vi "Stratified KFold Indices.vi"(8 "error in (no error)":errorcluster, 9 "seed":i32=-1 caption="seed (-1)", 10 "Nr Folds":i32=10 caption="Nr Folds (10)", 11 "Labels y":dbl[](array[numeric])) -> (0 "error out":errorcluster, 3 "Stratified KFold indices":cluster{"elements":i32[]}[](array[cluster]))   [LabVIEW 2014]
uses:
  <userlib>/_OpenG.lib/array/array.llb/Index 1D Array Elements (I32)__ogtk.vi
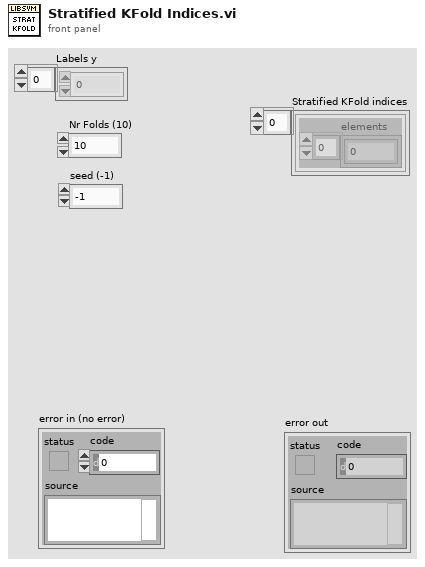
[diagram p1: front panel]
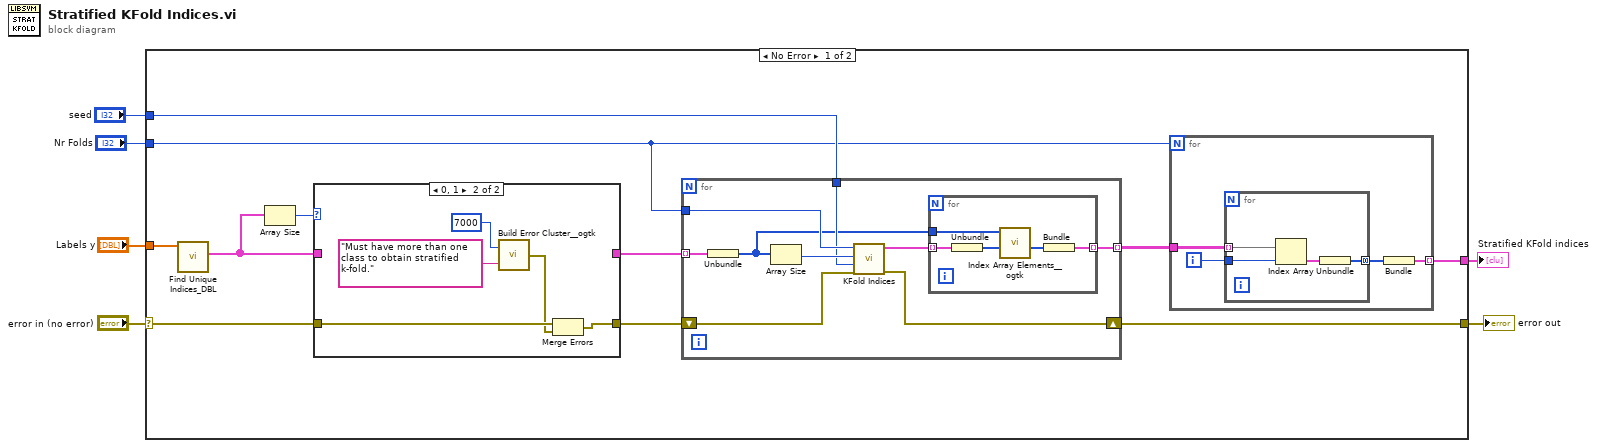
[diagram p0: block diagram]
diagram:
  n1 = case shown="No Error" "error in (no error)" {
    selector: "error in (no error)" -> [w14 w47]
    tunnel: [w8 w47] -> w3
    tunnel: "Labels y" -> [w17 _]
    tunnel: "Nr Folds" -> [w10 _]
    tunnel: "seed" -> [w12 _]
    tunnel: [w7 _] -> w1
    frame No Error {
      n2 = call "Find Unique Indices_DBL.vi"("Input Array"=w17) -> ("Unique indices"=w15:cluster{i32[]}[])  [unwired: 9 in, 1 out]
      n3 = Array Size(array=w15) -> (size(s)=w16:i32)
      n4 = case shown="0, 1" w16 {
        tunnel: w15 -> [w40 _]
        tunnel: w14 -> [w41 w44]
        tunnel: [w41 w42] -> w13
        tunnel: [w40 _] -> w11
        frame Default {
        }
        frame 0, 1 {
          n5 = call <userlib>:"Build Error Cluster__ogtk.vi"("String to Prepend to source (\"\")"="Must have more than one class to obtain stratified k-fold." ("String to Prepend to source (\"\")"), "code"=7000) -> ("error out"=w43:errorcluster)
          n6 = Merge Errors(w44, w43) -> (w42:errorcluster)
        }
      }
      n7 = for {
        tunnel: w11 -> [w34] mode=indexing
        tunnel: w10 -> [w32]
        shift-right: [w31] -> w8
        shift-left: w13 -> [w30]
        tunnel: w12 -> [w29]
        tunnel: [w26] -> w9 mode=indexing
        n8 = Unbundle(w34) -> (w27:i32[])
        n9 = Array Size(array=w27) -> (size(s)=w33:i32)
        n10 = call "KFold Indices.vi"("error in (no error)"=w30, "seed"=w29, "Data size"=w33, "Nr Folds"=w32) -> ("error out"=w31:errorcluster, "Fold indices"=w28:cluster{i32[]}[])  [unwired: 6 in]
        n11 = for {
          tunnel: w28 -> [w39] mode=indexing
          tunnel: w27 -> [w37]
          tunnel: [w35] -> w26 mode=indexing
          n12 = Unbundle(w39) -> (w38:i32[])
          n13 = call-poly <userlib>:"Index Array Elements__ogtk.vi"("indices"=w38, "array"=w37) -> ("elements"=w36:i32[])  [unwired: 9 in]
          n14 = Bundle("elements"=w36) -> (w35:cluster{"elements":i32[]})  [unwired: 1 in]
        }
      }
      n15 = for {
        N: w10 -> [_]
        tunnel: w9 -> [w21]
        tunnel: [w18] -> w7 mode=indexing
        i -> [w20]
        n16 = for {
          tunnel: w21 -> [w25] mode=indexing
          tunnel: w20 -> [w24]
          tunnel: [w22] -> w19 mode=concatenating
          n17 = Index Array(array=w25, index=w24) -> (element=w23:cluster{"elements":i32[]})
          n18 = Unbundle(w23) -> ("elements"=w22:i32[])
        }
        n19 = Bundle("elements"=w19) -> (w18:cluster{"elements":i32[]})  [unwired: 1 in]
      }
    }
    frame Error {
    }
  }
  "error out" <- w3
  "Stratified KFold indices" <- w1
